vi "Build Data Blocks.vi"(7 "reset? (F)":bool, 8 "error in (no error)":errorcluster, 9 "samples per cycle (192)":u16=192, 10 "cycles per block (10)":u16=10, 11 "resampled data":T1[](array[typedef]) {"resampled signal" format="%.2f"; "times [s]" format="%.2f"}) -> (0 "error out":errorcluster, 3 "data blocks":T1[][](array[typedef]) {"resampled signal" format="%.2f"; "times [s]" format="%.2f"})   [LabVIEW 2014, in "NI_EP_Power Measurement.lvlib"]
doc: "Builds even-angle-spaced voltage and current signals into data blocks."
uses:
  <vilib>/addons/Electrical Power/Power Measurement/NI_EP_Power Measurement.lvlib
  <vilib>/addons/Electrical Power/Power Measurement/subVIs/ep_Resampled Data.ctl
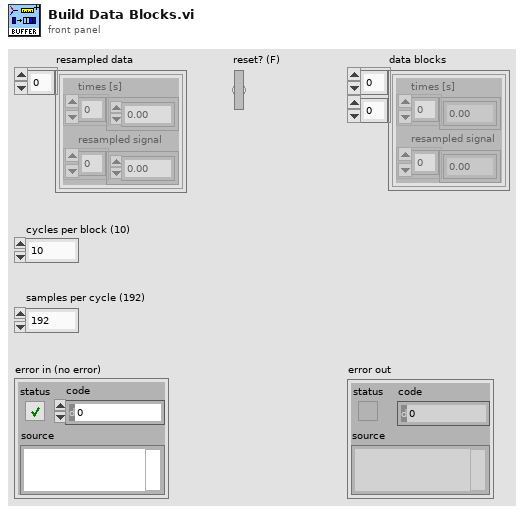
[diagram p1: front panel]
types:
  T1 = typedef "NI_EP_Power Measurement.lvlib/ep_Resampled Data.ctl" = cluster{"times [s]":dbl[], "resampled signal":dbl[]}
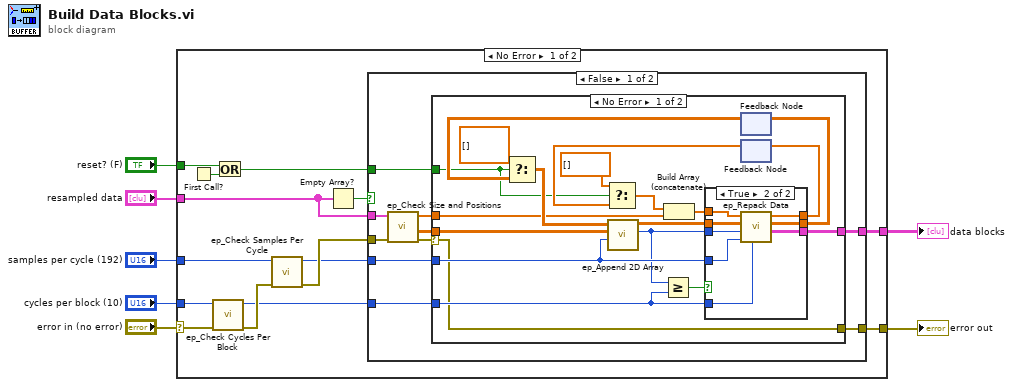
[diagram p0: block diagram]
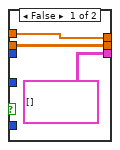
[diagram p2: hidden frame]
diagram:
  n1 = case shown="No Error" "error in (no error)" {
    selector: "error in (no error)" -> [w11 w64]
    tunnel: "cycles per block (10)" -> [w12 _]
    tunnel: "samples per cycle (192)" -> [w10 _]
    tunnel: "reset? (F)" -> [w20 _]
    tunnel: "resampled data" -> [w17 _]
    tunnel: [w19 _] -> w4
    tunnel: [w16 w64] -> w1
    frame No Error {
      n2 = First Call?() -> (First Call?: T/F=w21:bool)
      n3 = call <vilib>:"ep_Check Cycles Per Block.vi"("error in (no error)"=w11, "cycles per block"=w12) -> ("error out"=w13:errorcluster, "dup cycles per block"=w9:u16)  [unwired: 8 in]
      n4 = Or(x=w20, y=w21) -> (x .or. y?=w18:bool)
      n5 = call <vilib>:"ep_Check Samples Per Cycle.vi"("error in (no error)"=w13, "samples per cycle"=w10) -> ("error out"=w14:errorcluster, "dup samples per cycle"=w8:u16)  [unwired: 8 in]
      n6 = Empty Array?(array=w17) -> (empty?=w15:bool)
      n7 = case shown="False" w15 {
        tunnel: w8 -> [w30 _]
        tunnel: w9 -> [w31 _]
        tunnel: [w29 _] -> w19
        tunnel: w18 -> [w28 _]
        tunnel: w17 -> [w25 _]
        tunnel: w14 -> [w24 w63]
        tunnel: [w22 w63] -> w16
        frame False {
          n8 = call <vilib>:"ep_Check Size and Positions.vi"("error in (no error)"=w24, "resampled data"=w25) -> ("error out"=w23:errorcluster, "resampled signal"=w26:dbl[][], "positions [s]"=w27:dbl[])  [unwired: 7 in]
          n9 = case shown="No Error" w23 {
            selector: w23 -> [w32 w62]
            tunnel: w31 -> [w50 _]
            tunnel: w30 -> [w49 _]
            tunnel: [w44 _] -> w29
            tunnel: w28 -> [w35 _]
            tunnel: w27 -> [w34 _]
            tunnel: w26 -> [w33 _]
            tunnel: [w32 w62] -> w22
            frame No Error {
              n10 = feedback #1() -> (w37:dbl[][])  [unwired: 1 in]
              n11 = Select(t=dbl[][] [] ("remained signal"), s=w35, f=w37) -> (s? t:f=w36:dbl[][])
              n12 = call <vilib>:"ep_Append 2D Array.vi"("samples per cycle"=w49, "current data"=w33, "history data"=w36) -> ("total cycles"=w41:i32, "appended data"=w40:dbl[][])  [unwired: 6 in, 1 out]
              n13 = Greater Or Equal?(x=w41, y=w50) -> (x >= y?=w42:bool)
              n14 = feedback #2() -> (w45:dbl[])  [unwired: 1 in]
              n15 = Select(t=dbl[] [] ("remained signal"), s=w35, f=w45) -> (s? t:f=w46:dbl[])
              n16 = Build Array (concatenate)(w46, w34) -> (w43:dbl[])
              n17 = case shown="True" w42 {
                tunnel: w50 -> [_ w58]
                tunnel: w41 -> [_ w61]
                tunnel: w40 -> [w51 w55]
                tunnel: w43 -> [w52 w54]
                tunnel: w49 -> [_ w59]
                tunnel: [w51 w57] -> w39
                tunnel: [T1[][] [] ("data blocks") w60] -> w44
                tunnel: [w52 w56] -> w48
                frame False {
                }
                frame True {
                  n18 = call <vilib>:"ep_Repack Data.vi"("cycles per block"=w58, "samples per cycle"=w59, "total cycles"=w61, "appended data"=w55, "time positions in [s]"=w54) -> ("data blocks"=w60:T1[][], "remained data"=w57:dbl[][], "time positions out [s]"=w56:dbl[])  [unwired: 4 in]
                }
              }
              n19 = feedback-in #1(w39) -> ()
              n20 = feedback-in #2(w48) -> ()
            }
            frame Error {
            }
          }
        }
        frame True {
        }
      }
    }
    frame Error {
    }
  }
  "error out" <- w1
  "data blocks" <- w4
